vi "Data Sender.vi"(8 "error in (no error)":errorcluster, 10 "String To Send":string, 11 "VISA resource name":refnum<visa-resource-name>) -> (0 "error out":errorcluster, 3 "VISA resource name Out":refnum<visa-resource-name>)   [LabVIEW 2025]
uses:
  Globals/Cancelled Global.vi
  Globals/Percent Complete Global.vi
panel:
  out "Broken Up 64 Char Strings 2":string[](array[string])
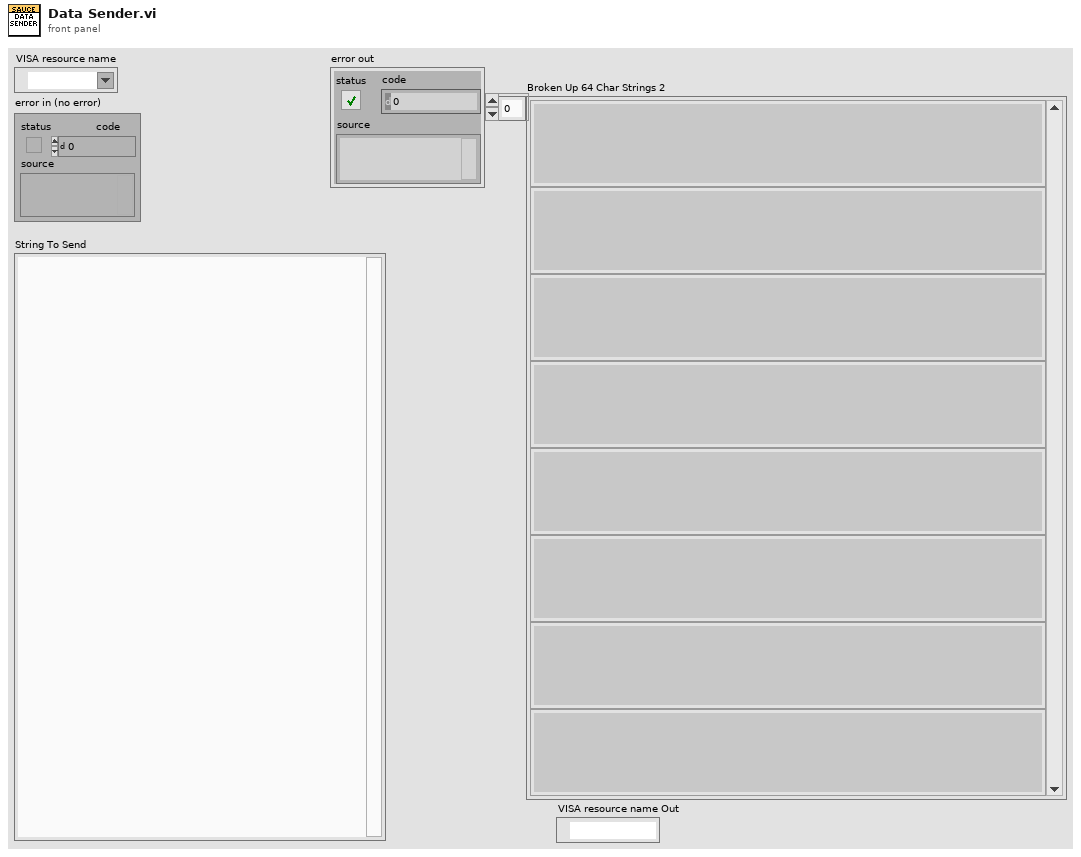
[diagram p1: front panel]
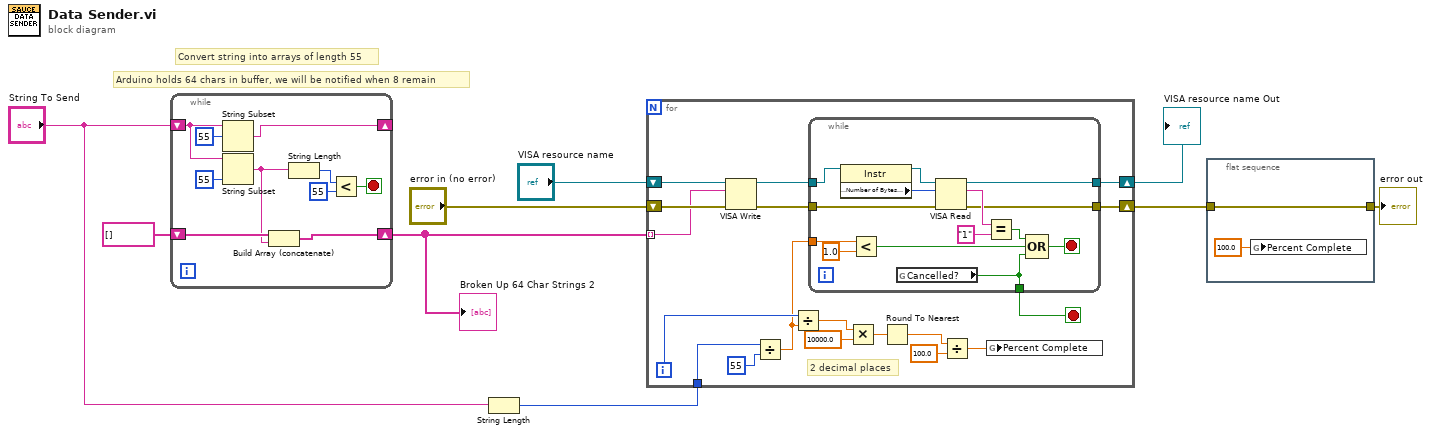
[diagram p0: block diagram]
diagram:
  # "Arduino holds 64 chars in buffer, we will be notified when 8 remain"
  # "Convert string into arrays of length 55"
  n1 = while {
    shift-right: [w11] -> _
    shift-left: "String To Send" -> [w15]
    shift-right: [w16] -> w8
    shift-left: string[] [] ("Broken Up 64 Char Strings") -> [w17]
    stop <- w14 stop-if-true
    n2 = String Subset(string=w15, offset (0)=55) -> (substring=w11:string)  [unwired: 1 in]
    n3 = String Subset(string=w15, length (rest)=55 ("length (rest)")) -> (substring=w10:string)  [unwired: 1 in]
    n4 = Build Array (concatenate)(w17, w10) -> (w16:string[])
    n5 = String Length(string=w10) -> (length=w12:i32)
    n6 = Less?(x=w12, y=55) -> (x < y?=w14:bool)
  }
  "Broken Up 64 Char Strings 2" <- w8
  n7 = String Length(string="String To Send") -> (length=w6:i32)
  n8 = for {
    tunnel: w8 -> [w35] mode=indexing
    shift-right: [w32] -> w1
    shift-left: "VISA resource name" -> [w37]
    shift-right: [w31] -> w2
    shift-left: "error in (no error)" -> [w36]
    tunnel: w6 -> [w27]
    i -> [w26]
    stop <- w30 stop-if-true
    # "2 decimal places"
    n9 = VISA Write(VISA resource name=w37, write buffer=w35, error in (no error)=w36) -> (VISA resource name out=w34:refnum<visa-resource-name>, error out=w33:errorcluster)  [unwired: 1 out]
    n10 = Divide(x=w27, y=55) -> (x/y=w20:dbl)
    n11 = Divide(x=w26, y=w20) -> (x/y=w25:dbl)
    n12 = while {
      tunnel: w34 -> [w51]
      tunnel: w33 -> [w48]
      tunnel: [w45] -> w32
      tunnel: [w44] -> w31
      tunnel: [w42] -> w30
      tunnel: w20 -> [w40]
      stop <- w41 stop-if-true
      n13 = property class="Instr"(reference=w51) -> (reference out=w50:refnum<visa-resource-name>, "Serial Settings:Number of Bytes at Serial Port"=w49:u32)  [unwired: 1 in, 1 out]
      n14 = Less?(x=w40, y=1.0) -> (x < y?=w38:bool)
      n15 = global read "Cancelled Global.vi" "Cancelled?"() -> (w42:bool)
      n16 = VISA Read(VISA resource name=w50, byte count=w49, error in (no error)=w48) -> (VISA resource name out=w45:refnum<visa-resource-name>, read buffer=w47:string, error out=w44:errorcluster)  [unwired: 1 out]
      n17 = Equal?(x=w47, y="1") -> (x = y?=w43:bool)
      n18 = Compound Arithmetic op=OR(w43, w38, w42) -> (w41:bool)
    }
    n19 = Multiply(x=w25, y=10000.0) -> (x*y=w24:dbl)
    n20 = Round To Nearest(number=w24) -> (nearest integer value=w23:dbl)
    n21 = Divide(x=w23, y=100.0) -> (x/y=w21:dbl)
    n22 = global write "Percent Complete Global.vi" "Percent Complete"(w21) -> ()
  }
  "VISA resource name Out" <- w1
  n23 = flat-sequence {
    tunnel: w2 -> [w52]
    tunnel: [w52] -> w5
    frame #0 {
      n24 = global write "Percent Complete Global.vi" "Percent Complete"(100.0 ("Percent Complete")) -> ()
    }
  }
  "error out" <- w5
